vi "FiltroM1.vi"(10 "Numeric 3":dbl, 11 "Numeric in":dbl) -> (3 "Numeric out":dbl)   [LabVIEW 2017]
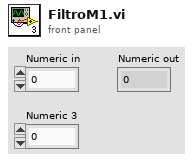
[diagram p1: front panel]
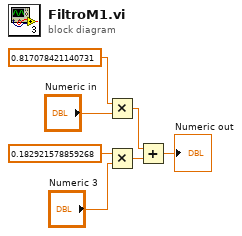
[diagram p0: block diagram]
diagram:
  n1 = Multiply(x=0.817078421140731, y="Numeric in") -> (x*y=w2:dbl)
  n2 = Multiply(x=0.182921578859268, y="Numeric 3") -> (x*y=w1:dbl)
  n3 = Add(x=w2, y=w1) -> (x+y=→"Numeric out":dbl)
